vi "Destroy Data.vi"(8 "error in (no error)":errorcluster, 11 "GRR Core in":refnum<class "GRR Core.lvclass">) -> (0 "error out":errorcluster, 3 "GRR Core out":refnum<class "GRR Core.lvclass">)   [LabVIEW 2018, in "GRR Core.lvclass"]
uses:
  GRR Core.lvclass
  GRR Core.lvclass/GRR Core.ctl
  TestDataMgr/TestDataMgr.lvclass
  Result Data Mgr/Result Data Mgr.lvclass
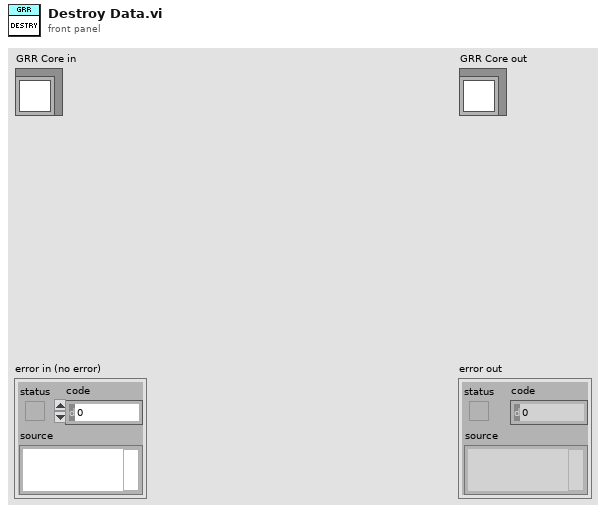
[diagram p1: front panel]
types:
  T1 = typedef "TestDataMgr.lvclass/Session Handle.ctl" = refnum<data-value>
  T2 = typedef "Result Data Mgr.lvclass/Session Handle.ctl" = refnum<data-value>
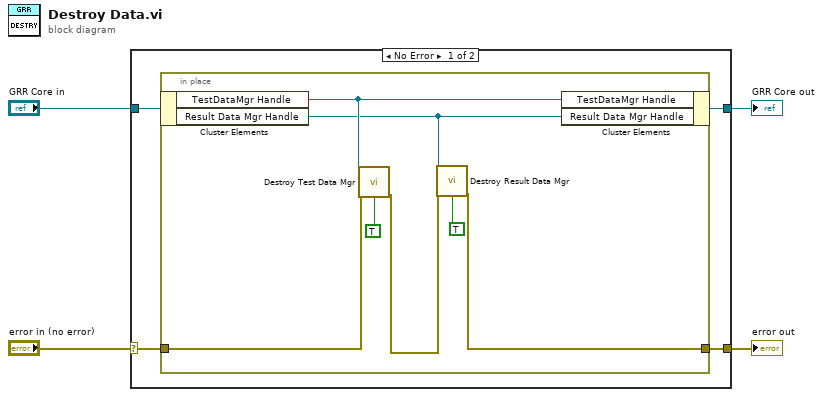
[diagram p0: block diagram]
diagram:
  n1 = case shown="No Error" "error in (no error)" {
    selector: "error in (no error)" -> [w6 w17]
    tunnel: [w5 w17] -> w3
    tunnel: [w7 w16] -> w1
    tunnel: "GRR Core in" -> [w8 w16]
    frame No Error {
      n2 = in-place {
        in-place-border: w6 -> [w15]
        in-place-border: [w11] -> w5
        n3 = in-place-cluster #1(w8) -> ("TestDataMgr Handle"=w10:T1, "Result Data Mgr Handle"=w9:T2)
        n4 = call "Destroy Test Data Mgr.vi"("Session Handle"=w10, "error in (no error)"=w15, "force destroy? (F)"=TRUE) -> ("error out"=w13:errorcluster)  [unwired: 12 in]
        n5 = call "Destroy Result Data Mgr.vi"("Session Handle"=w9, "error in (no error)"=w13, "force destroy? (F)"=TRUE) -> ("error out"=w11:errorcluster)  [unwired: 12 in]
        n6 = in-place-cluster #1("TestDataMgr Handle"=w10, "Result Data Mgr Handle"=w9) -> (w7:refnum<class "GRR Core.lvclass">)
      }
    }
    frame Error {
    }
  }
  "error out" <- w3
  "GRR Core out" <- w1
